vi "Refine triangles, random barycentric Delaunay.vi"(2 "Write STL file":bool, 3 "Refinement points per tri":i32=1, 4 "Refined STL file path":path, 5 "Original STL file path":path=path "C:/EnFlo Software/Anemometry/Utilities/Probe blockage potential flow sim/test stl files/Sphere.stl") -> (0 "N triangles after refinement":i32, 1 "N triangles before refinement":i32)   [LabVIEW 2017]
uses:
  <vilib>/Utility/miscctls.llb/LVRGBAColorTypeDef.ctl
  Anemometry Sub Vis/Collision_Detection/Triangles/Convex Hull/Typedefs/Triangle, indexed.ctl
  ctls/Triangle panel.ctl
  Anemometry Sub Vis/Collision_Detection/Triangles/Convex Hull/Subroutines/Creat unit normal.vi
  Anemometry Sub Vis/Collision_Detection/Triangles/Subroutines/Dot product.vi
  Anemometry Sub Vis/Collision_Detection/Triangles/Subroutines/Cross product 3D.vi
  Anemometry Sub Vis/Collision_Detection/Triangles/Subroutines/Unit vector.vi
panel:
  in  "Render mode":T1(ring)=enum."Wireframe"
  out "Refined STL view":refnum<vi>(3d-picture)
  out "Original STL view":refnum<vi>(3d-picture)
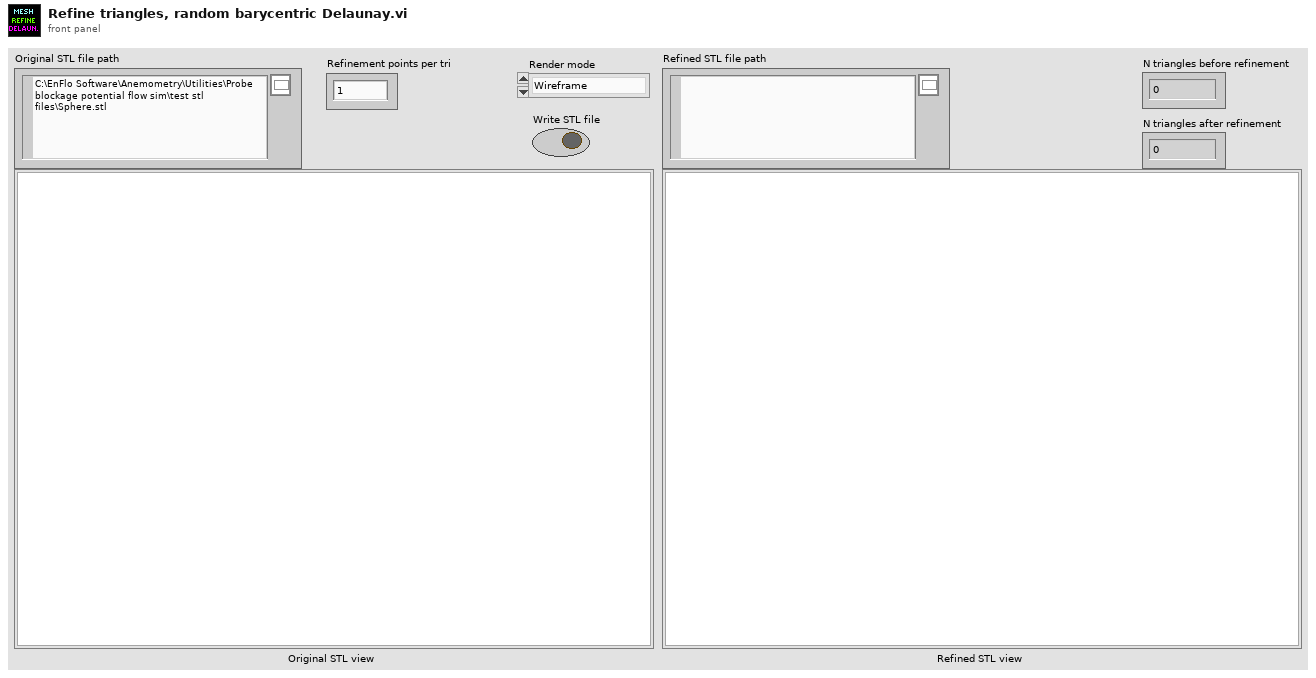
[diagram p1: front panel]
types:
  T1 = enum16{"Inherit Value", "Points", "Wireframe", "Polygons"}
  T2 = typedef "Triangle panel.ctl" = cluster{"V0":sgl[], "V1":sgl[], "V2":sgl[], "E0":sgl[], "E1":sgl[], "E2":sgl[], "n^":sgl[], "Pc":sgl[], "Gamma'":sgl, "V_transp.":sgl, "E0 link":i32, "E1 link":i32, "E2 link":i32}
  T3 = typedef "Triangle, indexed.ctl" = cluster{"V0":sgl[], "V1":sgl[], "V2":sgl[], "n^":sgl[], "i0":i32, "i1":i32, "i2":i32}
  T4 = typedef "LVRGBAColorTypeDef.ctl" = cluster{"Red":sgl, "Green":sgl, "Blue":sgl, "Alpha":sgl}
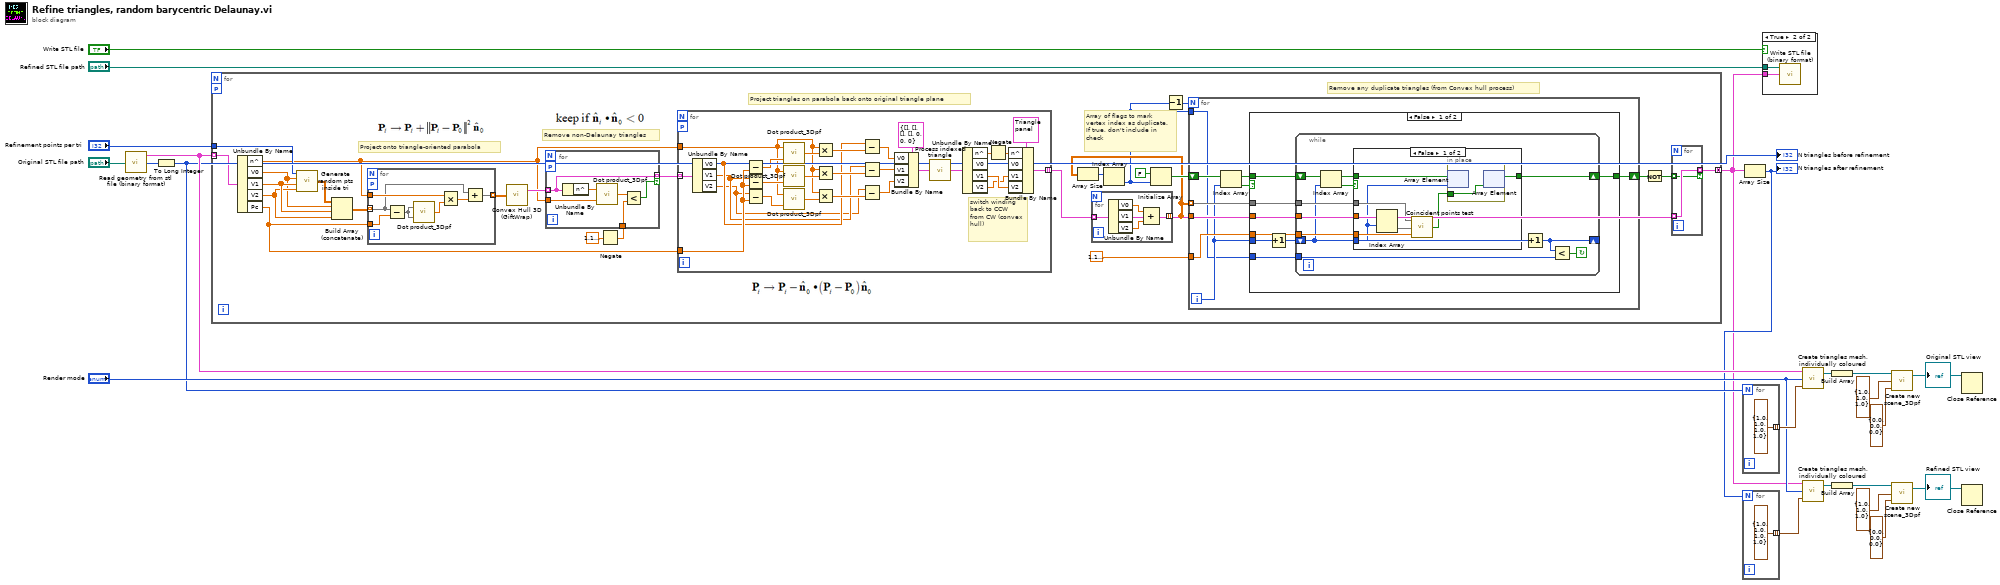
[diagram p0: block diagram]
diagram:
  n1 = call "Read geometry from stl file (binary format).vi"("STL file path"="Original STL file path") -> ("Panel triangles array"=w13:T2[], "N triangles"=w12:u32)  [unwired: 1 out]
  n2 = To Long Integer(number=w12) -> (32bit integer=w5:i32)
  "N triangles before refinement" <- w5
  n3 = for {
    tunnel: w13 -> [w47] mode=indexing
    workers-P: _ -> [_]
    tunnel: "Refinement points per tri" -> [w46]
    tunnel: [w26] -> w2 mode=concatenating
    # "Remove any duplicate triangles (from Convex hull process)"
    # "Project triangles on parabola back onto original triangle plane"
    # "Remove non-Delaunay triangles"
    # "Project onto triangle-oriented parabola"
    # "Array of flags to mark vertex index as duplicate. If true, don't include in check"
    n4 = Unbundle By Name(w47) -> ("n^"=w37:sgl[], "V0"=w39:sgl[], "V1"=w44:sgl[], "V2"=w43:sgl[], "Pc"=w36:sgl[])
    n5 = call "Generate random pts inside tri.vi"("V2"=w43, "V1"=w44, "V0"=w39, "N pts"=w46) -> ("Pts"=w45:sgl[][])
    n6 = Build Array (concatenate)(w45, w39, w44, w43) -> (w42:sgl[][])
    n7 = for {
      tunnel: w42 -> [w128] mode=indexing
      tunnel: w36 -> [w132]
      tunnel: w37 -> [w129]
      tunnel: [w126] -> w41 mode=indexing
      workers-P: _ -> [_]
      n8 = Subtract(x=w128, y=w132) -> (x-y=w131:sgl[])
      n9 = call "Dot product_3Dpf.vi"("B"=w131, "A"=w131) -> ("A . B"=w130:sgl)
      n10 = Multiply(x=w129, y=w130) -> (x*y=w127:sgl[])
      n11 = Add(x=w128, y=w127) -> (x+y=w126:sgl[])
    }
    n12 = call "Convex Hull 3D (GiftWrap).vi"("Vertices"=w41) -> ("Convex hull triangles, indexed"=w40:T3[])  [unwired: 1 out]
    n13 = Negate(x=sgl 1.1920929e-07) -> (-x=w34:sgl)
    n14 = for {
      tunnel: w40 -> [w123] mode=indexing
      tunnel: w37 -> [w124]
      tunnel: [w123] -> w38 mode=indexing if=w122
      workers-P: _ -> [_]
      tunnel: w34 -> [w120]
      n15 = Unbundle By Name(w123) -> ("n^"=w125:sgl[])
      n16 = call "Dot product_3Dpf.vi"("B"=w124, "A"=w125) -> ("A . B"=w121:sgl)
      n17 = Less?(x=w121, y=w120) -> (x < y?=w122:bool)
    }
    n18 = for {
      workers-P: _ -> [_]
      tunnel: w38 -> [w119] mode=indexing
      tunnel: w37 -> [w111]
      tunnel: w36 -> [w118]
      tunnel: [w98] -> w27 mode=indexing
      # "switch winding back to CCW from CW (convex hull)"
      n19 = Unbundle By Name(w119) -> ("V0"=w107:sgl[], "V1"=w106:sgl[], "V2"=w105:sgl[])
      n20 = Subtract(x=w107, y=w118) -> (x-y=w117:sgl[])
      n21 = Subtract(x=w106, y=w118) -> (x-y=w116:sgl[])
      n22 = Subtract(x=w105, y=w118) -> (x-y=w115:sgl[])
      n23 = call "Dot product_3Dpf.vi"("B"=w117, "A"=w111) -> ("A . B"=w114:sgl)
      n24 = call "Dot product_3Dpf.vi"("B"=w116, "A"=w111) -> ("A . B"=w112:sgl)
      n25 = call "Dot product_3Dpf.vi"("B"=w115, "A"=w111) -> ("A . B"=w113:sgl)
      n26 = Multiply(x=w111, y=w114) -> (x*y=w110:sgl[])
      n27 = Multiply(x=w111, y=w112) -> (x*y=w109:sgl[])
      n28 = Multiply(x=w111, y=w113) -> (x*y=w108:sgl[])
      n29 = Subtract(x=w107, y=w110) -> (x-y=w104:sgl[])
      n30 = Subtract(x=w106, y=w109) -> (x-y=w96:sgl[])
      n31 = Subtract(x=w105, y=w108) -> (x-y=w95:sgl[])
      n32 = Bundle By Name(cluster=T3 {"V0"=[], "V1"=[], "V2"=[], "n^"=[], "i0"=0, "i1"=0, "i2"=0} ("Triangle, indexed"), "V0"=w104, "V1"=w96, "V2"=w95) -> (w102:T3)
      n33 = call "Process indexed triangle.vi"("Triangle in (indexed)"=w102) -> ("Triangle out (indexed)"=w99:T3)
      n34 = Unbundle By Name(w99) -> ("n^"=w97:sgl[], "V0"=w100:sgl[], "V1"=w94:sgl[], "V2"=w93:sgl[])
      n35 = Negate(x=w97) -> (-x=w92:sgl[])
      n36 = Bundle By Name(cluster=T2 {"V0"=[], "V1"=[], "V2"=[], "E0"=[], "E1"=[], "E2"=[], "n^"=[], "Pc"=[], "Gamma'"=0.0, "V_transp."=0.0, "E0 link"=-1, "E1 link"=-1, "E2 link"=-1} ("Triangle Panel"), "n^"=w92, "V0"=w100, "V1"=w93, "V2"=w94) -> (w98:T2)
    }
    n37 = for {
      tunnel: w27 -> [w88] mode=indexing
      tunnel: [w87] -> w25 mode=indexing
      n38 = Unbundle By Name(w88) -> ("V0"=w91:sgl[], "V1"=w90:sgl[], "V2"=w89:sgl[])
      n39 = Compound Arithmetic op=ADD(w91, w90, w89) -> (w87:sgl[])
    }
    n40 = Array Size(array=w25) -> (size(s)=w30:i32[])
    n41 = Index Array(array=w30) -> (element=w23:i32)  [unwired: 1 in]
    n42 = Initialize Array(FALSE, w23) -> (w31:bool[])
    n43 = Decrement(x=w23) -> (x-1=w24:i32)
    n44 = for {
      N: w24 -> [_]
      tunnel: sgl 1.1920929e-07 -> [w57]
      tunnel: w25 -> [w56] mode=indexing
      shift-right: [w55] -> w32
      shift-left: w31 -> [w53]
      tunnel: w25 -> [w51]
      tunnel: w23 -> [w50]
      i -> [w54]
      n45 = Index Array(array=w53, index=w54) -> (element=w52:bool)
      n46 = case shown="False" w52 {
        tunnel: w57 -> [w64 _]
        tunnel: w54 -> [w63 _]
        tunnel: w56 -> [w62 _]
        tunnel: w51 -> [w58 _]
        tunnel: w50 -> [w61 _]
        tunnel: w53 -> [w60 w86]
        tunnel: [w59 w86] -> w55
        frame False {
          n47 = Increment(x=w63) -> (x+1=w65:i32)
          n48 = while {
            shift-right: [w67] -> _
            shift-left: w65 -> [w68]
            tunnel: w64 -> [w75]
            tunnel: w62 -> [w74]
            tunnel: w61 -> [w73]
            shift-right: [w71] -> w59
            shift-left: w60 -> [w70]
            tunnel: w58 -> [w66]
            stop <- w72 continue-if-true
            n49 = Index Array(array=w70, index=w68) -> (element=w69:bool)
            n50 = case shown="False" w69 {
              tunnel: w75 -> [w82 _]
              tunnel: w74 -> [w80 _]
              tunnel: w66 -> [w83 _]
              tunnel: w70 -> [w79 w85]
              tunnel: w68 -> [w78 _]
              tunnel: [w76 w85] -> w71
              frame False {
                n51 = Index Array(array=w83, index (row)=w78) -> (element=w81:sgl[])  [unwired: 1 in]
                n52 = call "Coincident points test.vi"("epsilon"=w82, "Point 2"=w81, "Point 1"=w80) -> ("Points are coincident"=w77:bool)
                n53 = in-place {
                  in-place-border: w77 -> [w84]
                  n54 = in-place-array #1(w79, w78) -> ()  [unwired: 1 out]
                  n55 = in-place-array #1(w84) -> (w76:bool[])  [unwired: 1 out]
                }
              }
              frame True {
              }
            }
            n56 = Increment(x=w68) -> (x+1=w67:i32)
            n57 = Less?(x=w67, y=w73) -> (x < y?=w72:bool)
          }
        }
        frame True {
        }
      }
    }
    n58 = Not(x=w32) -> (.not. x?=w33:bool[])
    n59 = for {
      tunnel: w27 -> [w49] mode=indexing
      tunnel: w33 -> [w48] mode=indexing
      tunnel: [w49] -> w26 mode=indexing if=w48
    }
  }
  n60 = for {
    N: w5 -> [_]
    tunnel: [T4 {"Red"=1.0, "Green"=1.0, "Blue"=1.0, "Alpha"=1.0} ("Colour")] -> w17 mode=indexing
  }
  n61 = Array Size(array=w2) -> (size(s)=w3:i32)
  "N triangles after refinement" <- w3
  n62 = for {
    N: w3 -> [_]
    tunnel: [T4 {"Red"=1.0, "Green"=1.0, "Blue"=1.0, "Alpha"=1.0} ("Colour")] -> w6 mode=indexing
  }
  n63 = case shown="True" "Write STL file" {
    tunnel: "Refined STL file path" -> [_ w136]
    tunnel: w2 -> [_ w135]
    frame False {
    }
    frame True {
      n64 = call "Write STL file (binary format).vi"("Panel triangles array"=w135, "STL file path"=w136) -> ()  [unwired: 2 in, 1 out]
    }
  }
  n65 = call "Create triangles mesh, individually coloured.vi"("Colours array"=w17, "Render mode"="Render mode", "Triangles array"=w13) -> ("Triangle mesh out"=w20:refnum<vi>)  [unwired: 1 out]
  n66 = call "Create triangles mesh, individually coloured.vi"("Colours array"=w6, "Render mode"="Render mode", "Triangles array"=w2) -> ("Triangle mesh out"=w8:refnum<vi>)  [unwired: 1 out]
  n67 = Build Array(w20) -> (w21:refnum<vi>[])
  n68 = Build Array(w8) -> (w9:refnum<vi>[])
  n69 = call "Create new scene_3Dpf.vi"("Translation"=cluster{"X":sgl, "Y":sgl, "Z":sgl} {"X"=0.0, "Y"=0.0, "Z"=0.0}, "Scale"=cluster{"X":sgl, "Y":sgl, "Z":sgl} {"X"=1.0, "Y"=1.0, "Z"=1.0}, "Scene objects array"=w21) -> ("Scene out"=w22:refnum<vi>)  [unwired: 1 out]
  "Original STL view" <- w22
  n70 = call "Create new scene_3Dpf.vi"("Translation"=cluster{"X":sgl, "Y":sgl, "Z":sgl} {"X"=0.0, "Y"=0.0, "Z"=0.0}, "Scale"=cluster{"X":sgl, "Y":sgl, "Z":sgl} {"X"=1.0, "Y"=1.0, "Z"=1.0}, "Scene objects array"=w9) -> ("Scene out"=w7:refnum<vi>)  [unwired: 1 out]
  "Refined STL view" <- w7
  n71 = Close Reference(reference=w22) -> ()  [unwired: 1 in, 1 out]
  n72 = Close Reference(reference=w7) -> ()  [unwired: 1 in, 1 out]
